vi "Remove Task In Map.vi"(8 "error in (no error)":errorcluster, 10 "Task ID":i64, 11 "Composite Map Task in":refnum<class "Composite Map Task.lvclass">) -> (0 "error out":errorcluster, 3 "Composite Map Task out":refnum<class "Composite Map Task.lvclass">)   [LabVIEW 2022 SP3, in "Composite Map Task.lvclass"]
uses:
  Composite Map Task.lvclass
  Composite Map Task.lvclass/Composite Map Task.ctl
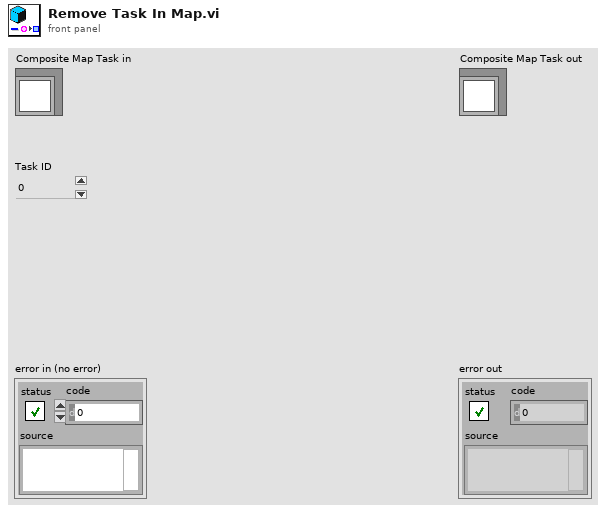
[diagram p1: front panel]
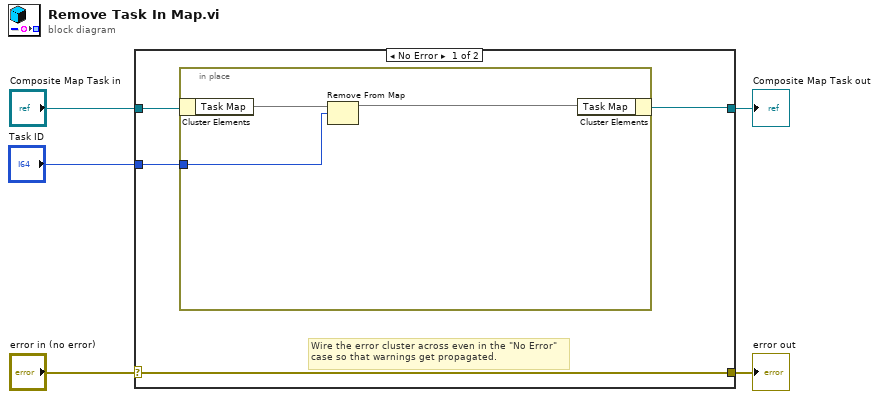
[diagram p0: block diagram]
diagram:
  n1 = case shown="No Error" "error in (no error)" {
    selector: "error in (no error)" -> [w9 w14]
    tunnel: [w9 w14] -> w4
    tunnel: [w7 w13] -> w2
    tunnel: "Composite Map Task in" -> [w8 w13]
    tunnel: "Task ID" -> [w6 _]
    frame No Error {
      # "Wire the error cluster across even in the \"No Error\"\ncase so that warnings get propagated."
      n2 = in-place {
        in-place-border: w6 -> [w10]
        n3 = in-place-cluster #1(w8) -> ("Task Map"=w12:map{i64, refnum<class "Task Ancestor.lvclass">})
        n4 = Remove From Map(10:w10, 11:w12) -> (3:w11:map{i64, refnum<class "Task Ancestor.lvclass">})  [unwired: 2 out]
        n5 = in-place-cluster #1("Task Map"=w11) -> (w7:refnum<class "Composite Map Task.lvclass">)
      }
    }
    frame Error {
    }
  }
  "error out" <- w4
  "Composite Map Task out" <- w2
